vi "Logger.ConvertStatusText.vi"(1 "Status string":string) -> (0 "Status":T1)   [LabVIEW 2016]
uses:
  Sequence/Sequence.Step.Status.ctl
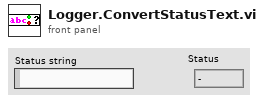
[diagram p1: front panel]
types:
  T1 = typedef "Sequence.Step.Status.ctl" = enum16{"-", "Pending", "Running", "Skipped", "Passed", "Failed", "Done", "Error", "Aborted", "Stopped"}
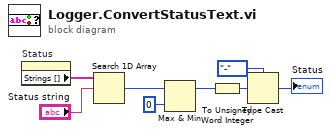
[diagram p0: block diagram]
diagram:
  n1 = property on="Status" class="Enum (strict)"() -> ("Strings []"=w2:string[])  [unwired: 2 in, 2 out]
  n2 = Search 1D Array(1D array=w2, element="Status string") -> (index of element=w6:i32)  [unwired: 1 in]
  n3 = Max & Min(x=w6, y=0) -> (max(x,y)=w5:i32)  [unwired: 1 out]
  n4 = To Unsigned Word Integer(number=w5) -> (unsigned 16bit integer=w8:u16)
  n5 = Type Cast(type=Sequence.Step.Status."-" ("_status"), x=w8) -> (*(type *) &x=→"Status":T1)
